vi "Valve Control Message Loop.vi"(8 "error in (no error)":errorcluster) -> (0 "error out":errorcluster)   [LabVIEW 2020, in "Valve Control.lvlib"]
doc: "Message loop for handling messages pertaining to the acquisition of data from the hardware."
uses:
  Valve Control.lvlib
  support/PCT FGV CMD.ctl
  Acquisition State.ctl
  AM Configuration.ctl
  support/Message Queue/Message Cluster.ctl
  support/Message Queue/Enqueue Message (Single).vi
  support/Message Queue/Message Queue.lvlib
  <vilib>/ErrorRing/Error Ring.xnode
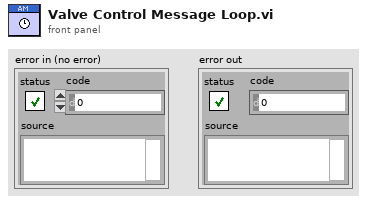
[diagram p1: front panel]
types:
  T1 = typedef "PCT FGV CMD.ctl" = enum16{"INIT", "GET", "SET"}
  T2 = typedef "PCT Data REFs.ctl" = cluster{"PLC AI Notifier":refnum<notifier>, "PS Data Queue":refnum<queue>, "BTN Queue":refnum<queue>, "PLC DI notifier":refnum<notifier>, "Timer notifier":refnum<notifier>, "DMM PS":refnum<notifier>, "DMM Gages":refnum<notifier>, "XYZ notifier":refnum<notifier>, "Test Notifier":refnum<notifier>, "Scanner notifier":refnum<notifier>, "OPC Notifier":refnum<notifier>, "HIDEN queue":refnum<queue>}
  T3 = typedef "Message Queue.lvlib/All Message Queues.ctl" = cluster{"UI":refnum<queue>, "Logging":refnum<queue>, "LOG":refnum<queue>, "ALARM":refnum<queue>, "Test":refnum<queue>, "Answer":refnum<queue>, "PLC":refnum<queue>, "DB":refnum<queue>, "Report":refnum<queue>, "OPC":refnum<queue>, "Procedure":refnum<queue>, "PalmSens":refnum<queue>, "SYS 7000 Reader":refnum<queue>, "SWITCH":refnum<queue>, "MOTOR":refnum<queue>, "MOTION":refnum<queue>, "HIDEN":refnum<queue>, "VALVE":refnum<queue>, "MFC":refnum<queue>, "PUMP IN":refnum<queue>, "PUMP OUT":refnum<queue>}
  T4 = typedef "Valve Control.lvlib/AM Configuration.ctl" = cluster{"Wait":dbl, "Next Step":string, "Writer Queue":refnum<queue>, "Reset":bool, "VISA resource":refnum<visa-resource-name>, "Status":bool[], "Valve Time":dbl[], "Timer queue":refnum<queue>, "Current valve":i32, "Enable":bool}
  T5 = typedef "Valve Control.lvlib/Acquisition State.ctl" = enum16{"Idle", "Initialized"}
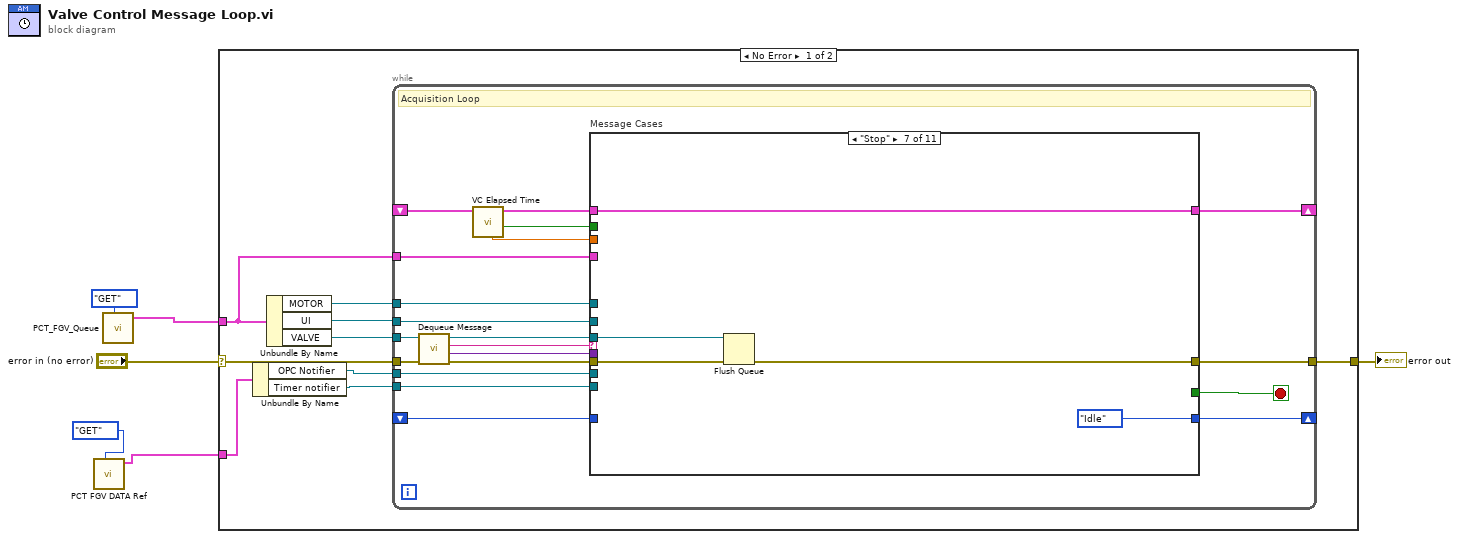
[diagram p0: block diagram]
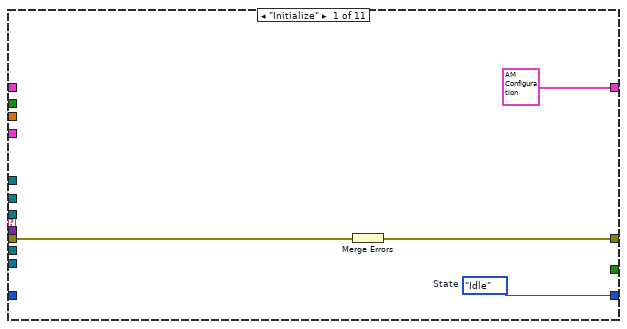
[diagram p2: hidden frame]
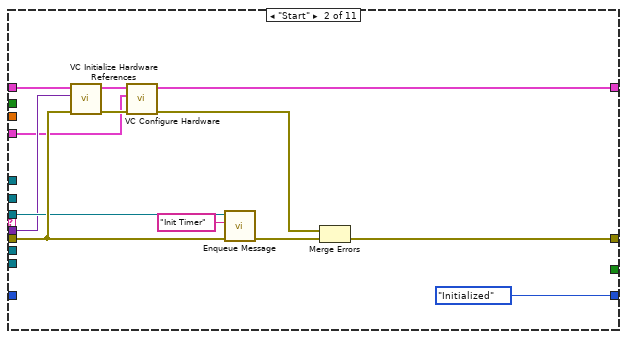
[diagram p3: hidden frame]
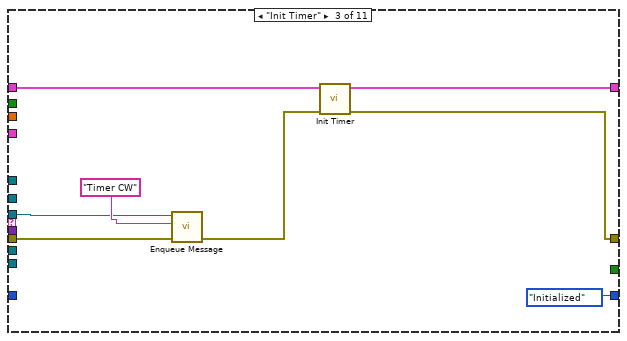
[diagram p4: hidden frame]
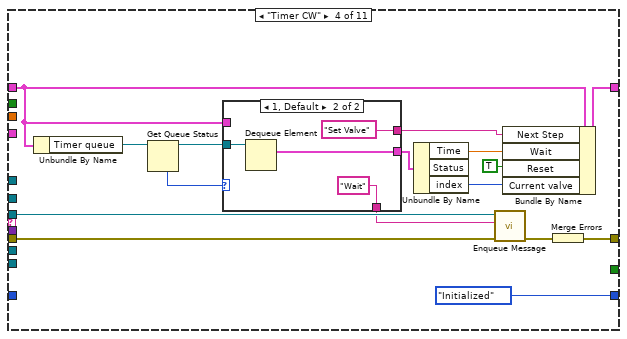
[diagram p5: hidden frame]
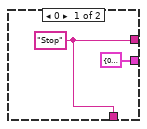
[diagram p6: hidden frame]
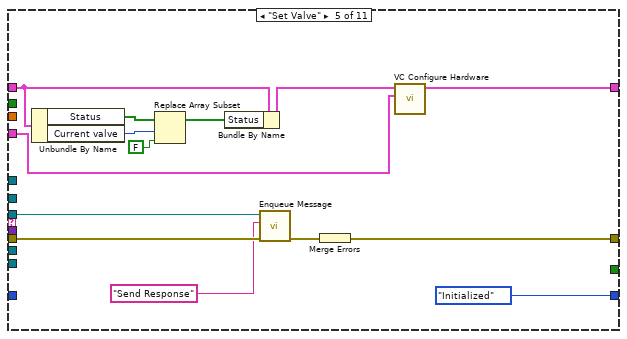
[diagram p7: hidden frame]
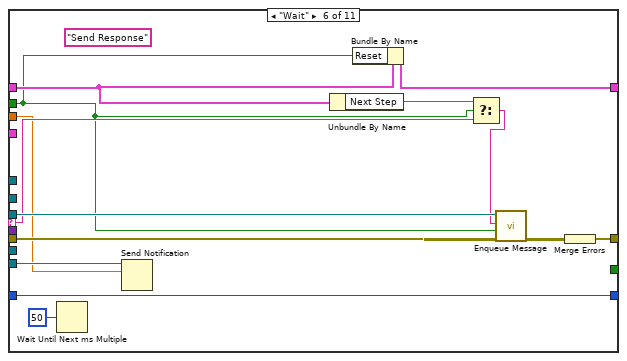
[diagram p8: hidden frame]
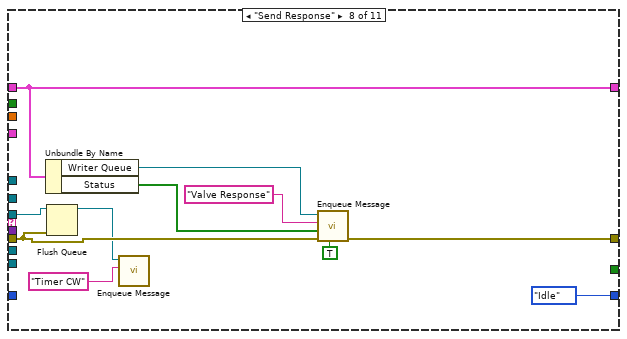
[diagram p9: hidden frame]
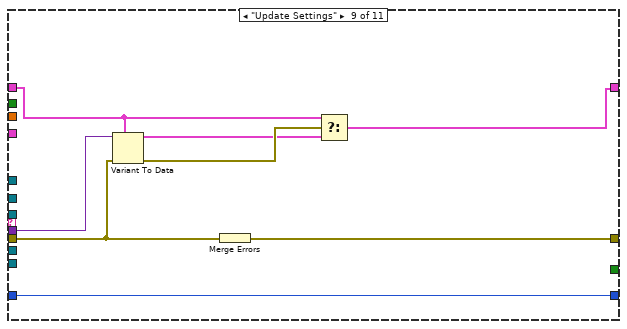
[diagram p10: hidden frame]
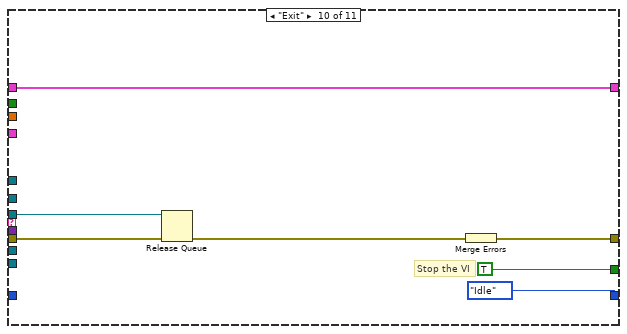
[diagram p11: hidden frame]
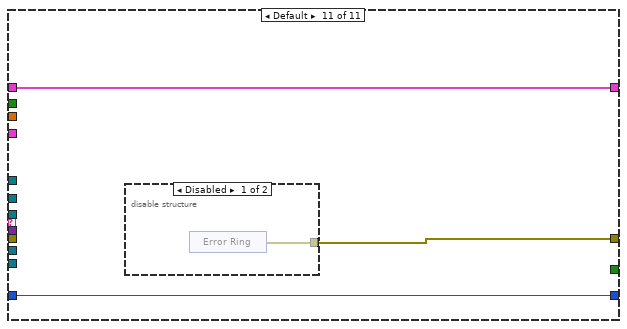
[diagram p12: hidden frame]
diagram:
  n1 = call "PCT FGV DATA Ref.vi"("CMD"=PCT_FGV_CMD."GET") -> ("Data REF"=w3:T2)  [unwired: 9 in, 1 out]
  n2 = call "PCT_FGV_Queue.vi"("CMD"=PCT_FGV_CMD."GET") -> ("Message Queues out"=w1:T3)  [unwired: 9 in, 1 out]
  n3 = case shown="No Error" "error in (no error)" {
    selector: "error in (no error)" -> [w13 w146]
    tunnel: w1 -> [w11 _]
    tunnel: [w14 w146] -> w6
    tunnel: w3 -> [w10 _]
    frame No Error {
      n4 = Unbundle By Name(w10) -> ("OPC Notifier"=w7:refnum<notifier>, "Timer notifier"=w9:refnum<notifier>)
      n5 = Unbundle By Name(w11) -> ("MOTOR"=w8:refnum<queue>, "UI"=w12:refnum<queue>, "VALVE"=w15:refnum<queue>)
      n6 = while {
        tunnel: w15 -> [w29]
        shift-right: [w35] -> _
        shift-left: _ -> [w18]
        tunnel: w12 -> [w25]
        shift-right: [w27] -> _
        shift-left: _ -> [w28]
        tunnel: w11 -> [w21]
        tunnel: w13 -> [w33]
        tunnel: [w19] -> w14
        tunnel: w9 -> [w20]
        tunnel: w8 -> [w17]
        tunnel: w7 -> [w16]
        stop <- w34 stop-if-true
        # "Acquisition Loop"
        n7 = call "Dequeue Message.vi"("error in (no error)"=w33, "Message Queue"=w29) -> ("error out"=w32:errorcluster, "Message Data"=w30:variant, "Message"=w31:string, "dup Message Queue"=w26:refnum<queue>)  [unwired: 6 in]
        n8 = call "VC Elapsed Time.vi"("AM Refs in"=w18) -> ("Time has Elapsed"=w23:bool, "AM Refs in"=w24:T4, "Elapsed Time (s)"=w22:dbl)  [unwired: 8 in]
        n9 = case "Message Cases" shown="\"Stop\"" w31 {
          selector: w31 -> [_ _ _ _ _ w101 _ _ _ _ _]
          tunnel: w26 -> [_ w49 w54 w73 w93 w105 w114 w121 _ w135 _]
          tunnel: w32 -> [w38 w50 w58 w74 w94 w106 w112 w118 w129 w137 _]
          tunnel: [w39 w52 w59 w75 w95 w108 w111 w125 w133 w139 w141] -> w19
          tunnel: w24 -> [_ w51 w53 w63 w86 w98 w110 w119 w127 w138 w143]
          tunnel: [T4 {"Wait"=0.0, "Next Step"="", "Writer Queue"=refnum, "Reset"=FALSE, "VISA resource"="", "Status"=[], "Valve Time"=[], "Timer queue"=refnum, "Current valve"=0, "Enable"=FALSE} ("Data Cluster") w48 w56 w70 w84 w102 w110 w119 w126 w138 w143] -> w35
          tunnel: [_ _ _ _ _ _ _ _ _ TRUE _] -> w34
          tunnel: w30 -> [_ w46 _ _ _ _ _ _ w132 _ _]
          tunnel: w25 -> [_ _ _ _ _ _ _ _ _ _ _]
          tunnel: w28 -> [_ _ _ _ _ w109 _ _ w128 _ w142]
          tunnel: [w37 Acquisition_State."Initialized" ("Acquisition State") Acquisition_State."Initialized" ("Acquisition State") Acquisition_State."Initialized" ("Acquisition State") Acquisition_State."Initialized" ("Acquisition State") w109 Acquisition_State."Idle" ("Acquisition State") Acquisition_State."Idle" ("Acquisition State") w128 Acquisition_State."Idle" ("Acquisition State") w142] -> w27
          tunnel: w23 -> [_ _ _ _ _ w96 _ _ _ _ _]
          tunnel: w22 -> [_ _ _ _ _ w99 _ _ _ _ _]
          tunnel: w21 -> [_ w40 _ _ w82 _ _ _ _ _ _]
          tunnel: w20 -> [_ _ _ _ _ w100 _ _ _ _ _]
          tunnel: w17 -> [_ _ _ _ _ _ _ _ _ _ _]
          tunnel: w16 -> [_ _ _ _ _ _ _ _ _ _ _]
          frame "Initialize" {
            w37 = Acquisition_State."Idle"  # State
            # "Initialize  - Initialize is currently a no-op.  The hardware initialization takes place in the 'Start' message."
            n10 = Merge Errors(w38) -> (w39:errorcluster)
          }
          frame "Start" {
            # "Start - Configure and start the acquisition."
            n11 = call "VC Initialize Hardware References.vi"("error in (no error)"=w50, "Message Data"=w46, "Hardware Resources in"=w51) -> ("error out"=w45:errorcluster, "Hardware Resources out"=w43:T4)  [unwired: 7 in]
            n12 = call "VC Configure Hardware.vi"("error in (no error)"=w45, "input cluster"=w40, "Hardware Resources in"=w43) -> ("error out"=w44:errorcluster, "Hardware Resources out"=w48:T4)  [unwired: 7 in]
            n13 = call-poly "Enqueue Message.vi"("error in (no error)"=w50, "Message"="Init Timer", "Message Queue"=w49) -> ("error out"=w42:errorcluster)  [unwired: 7 in, 1 out]
            n14 = Merge Errors(w44, w42) -> (w52:errorcluster)
          }
          frame "Init Timer" {
            # "Start - Configure and start the acquisition."
            n15 = call-poly "Enqueue Message.vi"("Message"="Timer CW", "Message Queue"=w54) -> ()  [unwired: 8 in, 2 out]
            n16 = call "Init Timer.vi"("error in (no error)"=w58, "AM Refs in in"=w53) -> ("error out"=w59:errorcluster, "AM Refs out"=w56:T4)  [unwired: 8 in]
          }
          frame "Timer CW" {
            # "Start - Configure and start the acquisition."
            n17 = Unbundle By Name(w63) -> ("Timer queue"=w69:refnum<queue>)
            n18 = Get Queue Status(queue=w69) -> (queue out=w67:refnum<queue>, # elements in queue=w68:i32)  [unwired: 2 in, 6 out]
            n19 = case shown="1, Default" w68 {
              tunnel: w67 -> [_ w81]
              tunnel: [cluster{"Time":dbl, "Status":bool, "index":i32} {"Time"=0.0, "Status"=FALSE, "index"=0} ("Timer Data") w80] -> w66
              tunnel: w63 -> [_ _]
              tunnel: [w76 "Set Valve" ("Message")] -> w62
              tunnel: [w76 "Wait" ("Message")] -> w61
              frame 0 {
                w76 = "Stop" ("Next Step")
              }
              frame 1, Default {
                n20 = Dequeue Element(queue=w81) -> (element=w80:cluster{"Time":dbl, "Status":bool, "index":i32})  [unwired: 2 in, 3 out]
              }
            }
            n21 = Unbundle By Name(w66) -> ("Time"=w65:dbl, "index"=w64:i32)  [unwired: 1 out]
            n22 = call-poly "Enqueue Message.vi"("error in (no error)"=w74, "Message"=w61, "Message Queue"=w73) -> ("error out"=w71:errorcluster)  [unwired: 7 in, 1 out]
            n23 = Bundle By Name(cluster=w63, "Next Step"=w62, "Wait"=w65, "Reset"=TRUE, "Current valve"=w64) -> (w70:T4)
            n24 = Merge Errors(w71) -> (w75:errorcluster)
          }
          frame "Set Valve" {
            # "Start - Configure and start the acquisition."
            n25 = Unbundle By Name(w86) -> ("Status"=w89:bool[], "Current valve"=w88:i32)
            n26 = Replace Array Subset(array=w89, new element=FALSE ("new element/subarray"), index=w88) -> (w85:bool[])
            n27 = Bundle By Name(cluster=w86, "Status"=w85) -> (w90:T4)
            n28 = call-poly "Enqueue Message.vi"("error in (no error)"=w94, "Message"="Send Response" ("Next Step"), "Message Queue"=w93) -> ("error out"=w91:errorcluster)  [unwired: 7 in, 1 out]
            n29 = Merge Errors(w91) -> (w95:errorcluster)
            n30 = call "VC Configure Hardware.vi"("input cluster"=w82, "Hardware Resources in"=w90) -> ("Hardware Resources out"=w84:T4)  [unwired: 8 in, 1 out]
          }
          frame "Wait" {
            (unwired) "Send Response" ("Next Step")
            # "Start - Configure and start the acquisition."
            n31 = Wait Until Next ms Multiple(millisecond multiple=u32 50) -> ()  [unwired: 1 out]
            n32 = Send Notification(notification=w99, notifier=w100) -> ()  [unwired: 1 in, 2 out]
            n33 = Unbundle By Name(w98) -> ("Next Step"=w97:string)
            n34 = Bundle By Name(cluster=w98, "Reset"=w96) -> (w102:T4)
            n35 = Select(t=w97, s=w96, f=w101) -> (s? t:f=w104:string)
            n36 = call-poly "Enqueue Message.vi"("error in (no error)"=w106, "Message Data"=w96, "Message"=w104, "Message Queue"=w105) -> ("error out"=w107:errorcluster)  [unwired: 6 in, 1 out]
            n37 = Merge Errors(w107) -> (w108:errorcluster)
          }
          frame "Stop" {
            # "Start - Configure and start the acquisition."
            n38 = Flush Queue(queue=w114, error in (no error)=w112) -> (error out=w111:errorcluster)  [unwired: 2 out]
          }
          frame "Send Response" {
            # "Acquire - Acquire data from the hardware. Since this is a continuous acquisition, this message will always message itself to run again."
            n39 = Unbundle By Name(w119) -> ("Writer Queue"=w124:refnum<queue>, "Status"=w117:bool[])
            n40 = Flush Queue(queue=w121, error in (no error)=w118) -> (queue out=w116:refnum<queue>)  [unwired: 2 out]
            n41 = call-poly "Enqueue Message.vi"("Message"="Timer CW", "Message Queue"=w116) -> ()  [unwired: 8 in, 2 out]
            n42 = call-poly "Enqueue Message.vi"("Priority Message? (F)"=TRUE, "error in (no error)"=w118, "Message Data"=w117, "Message"="Valve Response", "Message Queue"=w124) -> ("error out"=w125:errorcluster)  [unwired: 5 in, 1 out]
          }
          frame "Update Settings" {
            # "New settings are available, update the current ones stored in the shift register with the settings sent as part of the message"
            n43 = Variant To Data(error in=w129, type=w127, Variant=w132) -> (data=w130:T4, error out=w131:errorcluster)
            n44 = Merge Errors(w129) -> (w133:errorcluster)
            n45 = Select(t=w127, s=w131, f=w130) -> (s? t:f=w126:T4)
          }
          frame "Exit" {
            # "Stop the VI"
            # "Exit - Send the Exit message to the UI Message Handler."
            n46 = Release Queue(queue=w135, error in (no error)=w137) -> (error out=w136:errorcluster)  [unwired: 1 in, 2 out]
            n47 = Merge Errors(w136) -> (w139:errorcluster)
          }
          frame Default {
            # "'Default' case only runs if there is a message that isn't defined in any of the other cases.  Output a programming error."
            n48 = disable-structure shown="Disabled" {
              disable-tunnel: [w144 _] -> w141
              frame Disabled {
                n49 = xnode "Error Ring"() -> ("error out"=w144:errorcluster)
              }
              frame Enabled {
              }
            }
          }
        }
      }
    }
    frame Error {
    }
  }
  "error out" <- w6
